vi "Get MCP Gain Table.vi"(9 "pfPhotoepc":sgl, 10 "piGain":i32, 11 "iNum":i32) -> (1 "pfPhotoepc out":sgl, 2 "piGain out":i32, 3 "function return":u32)   [LabVIEW 2018, in "AndorSDK.lvlib"]
doc: "EXPNETTYPE unsigned int WINAPI GetMCPGainTable(int iNum, int * piGain, float * pfPhotoepc);"
uses:
  AndorSDK.lvlib
  ATMCD32D.dll
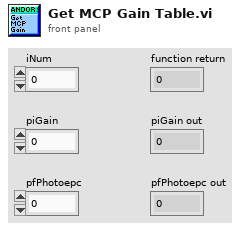
[diagram p1: front panel]
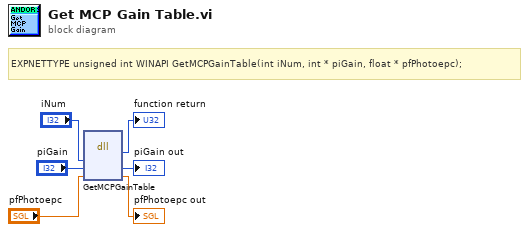
[diagram p0: block diagram]
diagram:
  # "EXPNETTYPE unsigned int WINAPI GetMCPGainTable(int iNum, int * piGain, float * pfPhotoepc);"
  n1 = dll-call lib="PTH2babs E\nPersönliches02 - Arbeit03-HiwijobsLabviewCodelibANDOR\tAndor SDK\nATMCD32D.*" fn="GetMCPGainTable"("iNum"="iNum", "piGain"="piGain", "pfPhotoepc"="pfPhotoepc") -> (→"function return":u32, "piGain"=→"piGain out":i32, "pfPhotoepc"=→"pfPhotoepc out":sgl)  [unwired: 4 in, 2 out]
